vi "SynchronizeTicklish.vi"(3 "error in (no error)":errorcluster, 5 "Serial USB port name":refnum<visa-resource-name>) -> (0 "error out":errorcluster, 1 "time-sync":T1, 2 "Serial USB port name out":refnum<visa-resource-name>)   [LabVIEW 2015]
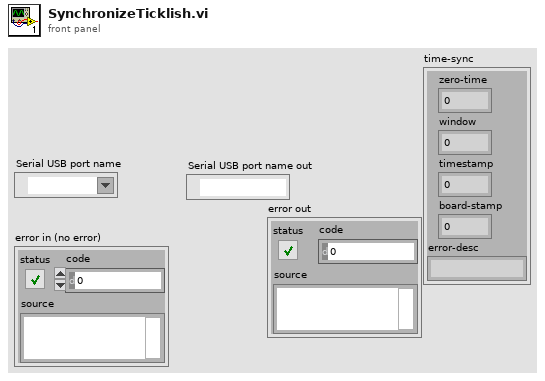
[diagram p1: front panel]
types:
  T1 = cluster{"zero-time":dbl, "window":dbl, "timestamp":dbl, "board-stamp":dbl, "error-desc":string}
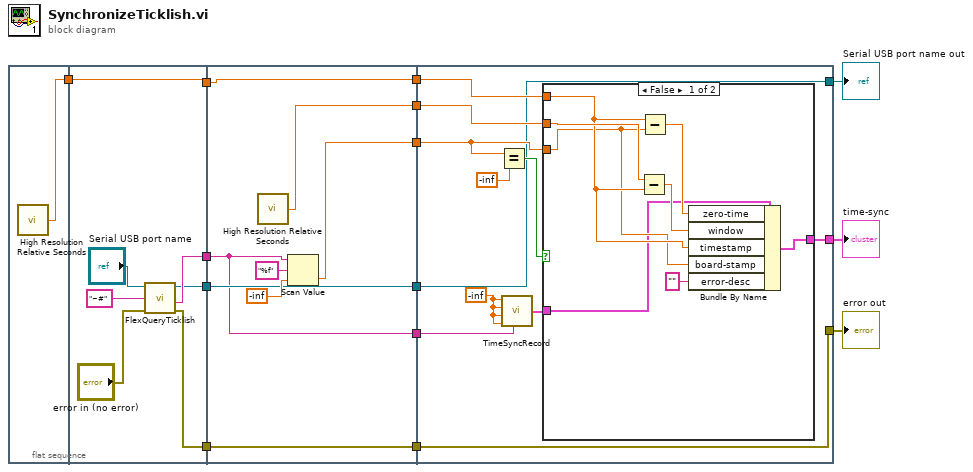
[diagram p0: block diagram]
diagram:
  n1 = flat-sequence {
    tunnel: [w15] -> w13
    tunnel: [w20] -> w14
    tunnel: w13 -> [w19]
    tunnel: [w19] -> w11
    tunnel: [w18] -> w7
    tunnel: [w17] -> w5
    tunnel: w14 -> [w23]
    tunnel: [w28] -> w12
    tunnel: w11 -> [w28]
    tunnel: [w27] -> w10
    tunnel: [w26] -> w9
    tunnel: [w25] -> w8
    tunnel: w7 -> [w25]
    tunnel: [w24] -> w6
    tunnel: w5 -> [w24]
    tunnel: [w23] -> w2
    tunnel: w12 -> [w39]
    tunnel: w10 -> [w38]
    tunnel: w9 -> [w37]
    tunnel: [w36] -> w3
    tunnel: w8 -> [w36]
    tunnel: [w35] -> w1
    tunnel: [w34] -> w4
    tunnel: w6 -> [w34]
    tunnel: w2 -> [w31]
    frame #0 {
      n2 = call <vilib>:"High Resolution Relative Seconds.vi"() -> ("relative seconds"=w15:dbl)
    }
    frame #1 {
      n3 = call "FlexQueryTicklish.vi"("error in (no error)"="error in (no error)", "write buffer"="~#", "Serial USB port name"="Serial USB port name") -> ("error out"=w18:errorcluster, "Result string"=w20:string, "Serial USB port name out"=w17:refnum<visa-resource-name>)  [unwired: 6 in]
    }
    frame #2 {
      n4 = call <vilib>:"High Resolution Relative Seconds.vi"() -> ("relative seconds"=w27:dbl)
      n5 = Scan Value(string=w23, format string="%f", default (0 dbl)=-inf) -> (value=w26:dbl)  [unwired: 1 out]
    }
    frame #3 {
      w33 = -inf
      n6 = Equal?(x=w37, y=-inf) -> (x = y?=w40:bool)
      n7 = call "TimeSyncRecord.vi"("zero-time"=w33, "window"=w33, "timestamp"=w33, "error-desc"=w31, "board-stamp"=w33) -> ("output cluster"=w32:T1)  [unwired: 3 in]
      n8 = case shown="False" w40 {
        tunnel: w39 -> [w46 _]
        tunnel: w38 -> [w49 _]
        tunnel: w37 -> [w45 _]
        tunnel: w32 -> [w44 w50]
        tunnel: [w43 w50] -> w35
        frame False {
          n9 = Subtract(x=w49, y=w46) -> (x-y=w47:dbl)
          n10 = Subtract(x=w46, y=w45) -> (x-y=w48:dbl)
          n11 = Bundle By Name(cluster=w44, "zero-time"=w48, "window"=w47, "timestamp"=w46, "board-stamp"=w45, "error-desc"="") -> (w43:T1)
        }
        frame True {
        }
      }
    }
  }
  "Serial USB port name out" <- w4
  "error out" <- w3
  "time-sync" <- w1
